vi "NS Cobra RT Launcher.vi"() -> ()   [LabVIEW 2019, in "Cobra RT.lvlib"]
uses:
  Cobra RT.lvlib
  Cobra RT/Cobra RT.lvclass
  C:/Program Files (x86)/National Instruments/LabVIEW 2019/vi.lib/ActorFramework/Actor/Actor.lvclass
  Cobra RT/Cobra RT.lvclass/Cobra RT.ctl
  <vilib>/NI/Actors/Network Endpoint Actors/Protocols/Network Stream Strategy/Netowrk Stream Listener/Network Stream Listener.lvclass
  C:/Program Files (x86)/National Instruments/LabVIEW 2019/vi.lib/ni/Actors/Network Endpoint Actors/Abstract Classes/Message Stream/Message Stream.lvclass
  <vilib>/ActorFramework/Actor/Actor.lvclass
  <vilib>/ni/Actors/Network Endpoint Actors/Protocols/Network Stream Strategy/Network Stream Initiator/Network Stream Initiator.lvclass
panel:
  in  "Initiator Name":string="Jung"
  in  "Address":string="127.0.0.1"
  in  "Listener Name":string="Stuart"
  # "Cobra"
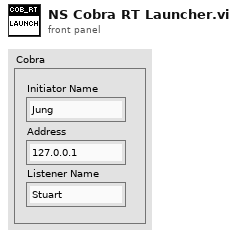
[diagram p1: front panel]
types:
  T1 = enum32{"Invalid", "Standard", "Closed", "Hidden", "Minimized", "Maximized"}
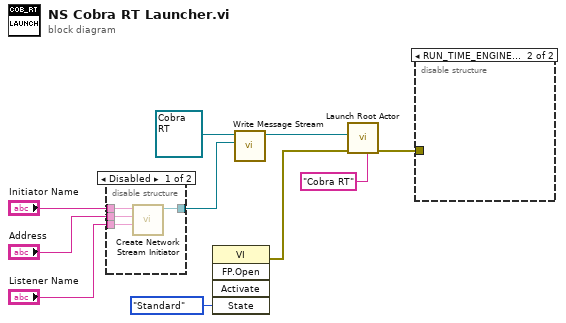
[diagram p0: block diagram]
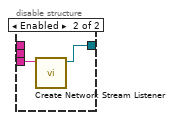
[diagram p2: hidden frame]
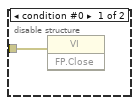
[diagram p3: hidden frame]
diagram:
  n1 = disable-structure shown="Disabled" {
    disable-tunnel: [w14 w15] -> w4
    disable-tunnel: "Initiator Name" -> [w13 _]
    disable-tunnel: "Address" -> [w12 _]
    disable-tunnel: "Listener Name" -> [w11 w16]
    frame Disabled {
      n2 = call <vilib>:"Create Network Stream Initiator.vi"("Remote Name"=w11, "Remote Address"=w12, "Name"=w13) -> ("Network Stream Initiator out"=w14:refnum<class "Network Stream Initiator.lvclass">)  [unwired: 8 in]
    }
    frame Enabled {
      n3 = call <vilib>:"Create Network Stream Listener.vi"("Name"=w16) -> ("Network Stream Listener"=w15:refnum<class "Network Stream Listener.lvclass">)  [unwired: 10 in]
    }
  }
  n4 = invoke class="VI" method="FP.Open"("State"=T1."Standard") -> (error out=w1:errorcluster)  [unwired: 4 in, 4 out]
  n5 = call "Write Message Stream.vi"("Message Stream"=w4, "Cobra RT In"=refnum<class "Cobra RT.lvclass"> refnum ("Cobra RT.lvlib:Cobra RT.lvclass")) -> ("Cobra RT Out"=w8:refnum<class "Cobra RT.lvclass">)  [unwired: 9 in]
  n6 = call <vilib>:"Launch Root Actor.vi"("Debug Alias"="Cobra RT", "error in (no error)"=w1, "Actor"=w8) -> ("error out"=w7:errorcluster)  [unwired: 7 in, 1 out]
  n7 = disable-structure shown="RUN_TIME_ENGINE==False" {
    disable-tunnel: w7 -> [w17 _]
    frame condition #0 {
      n8 = invoke class="VI" method="FP.Close"(error in=w17) -> ()  [unwired: 2 in, 3 out]
    }
    frame condition #1 (active) {
    }
  }
